vi "ma_Tone estimation (amplitude input).vi"(1 "spectral info":T1 {"window" items=["Rectangle"=0, "Hanning"=1, "Hamming"=2, "Blackman-Harris"=3, "Exact Blackman"=4, "Blackman"=5, "Flat Top"=6, "4 Term B-Harris "=7, "7 Term B-Harris"=8, "Low Sidelobe"=9, "Blackman Nuttall"=11, "Triangle"=30, "Bartlett-Hanning"=31, "Bohman"=32, "Parzen"=33, "Welch"=34, "Kaiser"=60, "Dolph-Chebyshev"=61, "Gaussian"=62]}, 2 "three fingers":T3={"f0"=0.0, "df"=1.0, "spectrum"=[]} {"spectrum" format="%.2f"; "df" format="%.2f"; "f0" format="%.2f"}) -> (0 "single tone info.":T2 {"phase [degree]" format="%.2f"; "amplitude" format="%.2f"; "frequency [Hz]" format="%.2f"})   [LabVIEW 2020, in "NI_MAPro.lvlib"]
doc: "This VI takes the three domainent FFT bins to apply the Newton-Raphson's root finding algorithm to determine the exact frequency, phase and amplitude.\nThe input is not necessary \"three fingers\", it could be two, four, or more."
uses:
  NI_MAPro.lvlib
  ma_sml_Spectrum Cluster (real).ctl
  ma_sml_Spectral Info.ctl
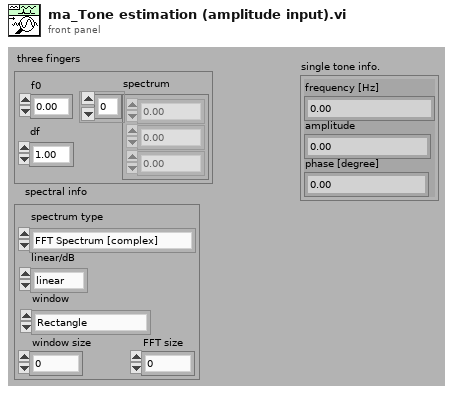
[diagram p1: front panel]
types:
  T1 = typedef "NI_MAPro.lvlib/ma_sml_Spectral Info.ctl" = cluster{"spectrum type":enum16{"FFT Spectrum [complex]", "Amplitude [Magnitude]", "Power [Magnitude^2]", "Cross Spectrum [complex]", "Frequency Response [Complex]"}, "linear/dB":enum16{"linear", "dB"}, "window":u16, "window size":i32, "FFT size":i32}
  T2 = cluster{"frequency [Hz]":dbl, "amplitude":dbl, "phase [degree]":dbl}
  T3 = typedef "NI_MAPro.lvlib/ma_sml_Spectrum Cluster (real).ctl" = cluster{"f0":dbl, "df":dbl, "spectrum":dbl[]}
  T4 = enum16{"FFT Spectrum [complex]", "Amplitude [Magnitude]", "Power [Magnitude^2]", "Cross Spectrum [complex]", "Frequency Response [Complex]"}
  T5 = cluster{"initial guess frequecy":dbl, "Amplitude":dbl, dbl}
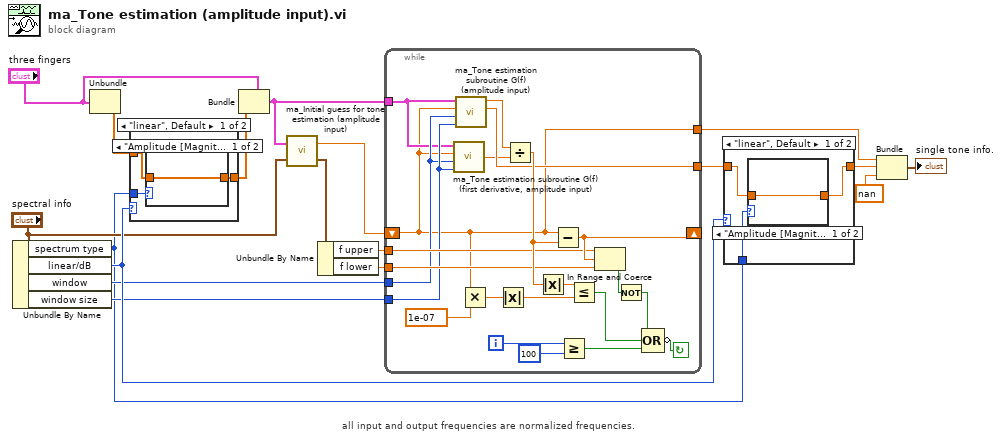
[diagram p0: block diagram]
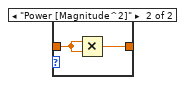
[diagram p2: hidden frame]
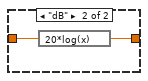
[diagram p3: hidden frame]
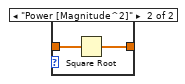
[diagram p4: hidden frame]
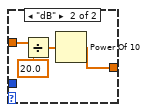
[diagram p5: hidden frame]
diagram:
  # "all input and output frequencies are normalized frequencies."
  n1 = Unbundle By Name("spectral info") -> ("spectrum type"=w2:T4, "linear/dB"=w13:enum16{"linear", "dB"}, "window"=w11:u16, "window size"=w10:i32)
  n2 = Unbundle("three fingers") -> ("spectrum"=w3:dbl[])  [unwired: 2 out]
  n3 = case shown="\"linear\", Default" w13 {
    tunnel: w3 -> [w20 w28]
    tunnel: [w19 w25] -> w6
    tunnel: w2 -> [w21 _]
    frame "linear", Default {
      n4 = case shown="\"Amplitude [Magnitude]\", Default" w21 {
        tunnel: [w22 w23] -> w19
        tunnel: w20 -> [w22 w24]
        frame "Amplitude [Magnitude]", Default {
        }
        frame "Power [Magnitude^2]" {
          n5 = Square Root(x=w24) -> (sqrt(x)=w23:dbl[])
        }
      }
    }
    frame "dB" {
      n6 = Divide(x=w28, y=20.0) -> (x/y=w26:dbl[])
      n7 = Power Of 10(x=w26) -> (10^x=w25:dbl[])
    }
  }
  n8 = Bundle(cluster="three fingers", "spectrum"=w6) -> (w5:T3)  [unwired: 2 out]
  n9 = call "ma_Initial guess for tone estimation (amplitude input).vi"("spectral info"="spectral info", "three fingers"=w5) -> ("range"=w9:cluster{"f upper":dbl, "f lower":dbl}, "initial guess frequecy"=w18:dbl)
  n10 = Unbundle By Name(w9) -> ("f upper"=w8:dbl, "f lower"=w7:dbl)
  n11 = while {
    tunnel: w7 -> [w38]
    tunnel: w8 -> [w39]
    tunnel: w10 -> [w37]
    tunnel: w11 -> [w36]
    tunnel: [w44] -> w15
    tunnel: [w32] -> w4
    shift-left: w18 -> [w32]
    shift-right: [w42] -> _
    tunnel: w5 -> [w35]
    i -> [w45]
    stop <- w47 continue-if-true
    n12 = call "ma_Tone estimation subroutine G(f) (first derivative, amplitude input).vi"("N (window length)"=w37, "window"=w36, "frequency"=w32, "three fingers"=w35) -> ("G'(f)"=w34:dbl)
    n13 = call "ma_Tone estimation subroutine G(f) (amplitude input).vi"("N (window length)"=w37, "window"=w36, "frequency"=w32, "three fingers"=w35) -> ("Amplitude"=w44:dbl, "G(f)"=w40:dbl)  [unwired: 2 in]
    n14 = Multiply(x=w32, y=1e-07) -> (x*y=w31:dbl)
    n15 = Absolute Value(x=w31) -> (abs(x)=w29:dbl)
    n16 = Divide(x=w40, y=w34) -> (x/y=w46:dbl)
    n17 = Absolute Value(x=w46) -> (abs(x)=w49:dbl)
    n18 = Subtract(x=w32, y=w46) -> (x-y=w42:dbl)
    n19 = Greater Or Equal?(x=w45, y=100) -> (x >= y?=w48:bool)
    n20 = Less Or Equal?(x=w49, y=w29) -> (x <= y?=w43:bool)
    n21 = In Range and Coerce(upper limit=w39, x=w42, lower limit=w38) -> (In Range?=w41:bool)  [unwired: 1 out]
    n22 = Not(x=w41) -> (.not. x?=w33:bool)
    n23 = Compound Arithmetic op=OR(w33, w43, w48) -> (invert w47:bool)
  }
  n24 = case shown="\"linear\", Default" w13 {
    tunnel: w15 -> [w52 w58]
    tunnel: [w51 w57] -> w14
    tunnel: w2 -> [w53 _]
    frame "linear", Default {
      n25 = case shown="\"Amplitude [Magnitude]\", Default" w53 {
        tunnel: [w54 w56] -> w51
        tunnel: w52 -> [w54 w55]
        frame "Amplitude [Magnitude]", Default {
        }
        frame "Power [Magnitude^2]" {
          n26 = Multiply(x=w55, y=w55) -> (x*y=w56:dbl)
        }
      }
    }
    frame "dB" {
      n27 = expression code="20*log(x)"(w58) -> (w57:dbl)
    }
  }
  n28 = Bundle("initial guess frequecy"=w4, "Amplitude"=w14, nan) -> (→"single tone info.":T5)  [unwired: 1 out]
